vi "ReadButtonUniques.vi"(8 "Error In":errorcluster, 11 "object in":refnum<class "TAFConfiguration.lvclass">) -> (0 "Error Out":errorcluster, 2 "ButtonUniques":T1, 3 "object out":refnum<class "TAFConfiguration.lvclass">)   [LabVIEW 2021, in "TAF Proj Document Type.lvlib" / "TAFConfiguration.lvclass"]
uses:
  <vilib>/Wovalab/AntiDoc/Document Type/Add-ons/LabVIEW TAF Project/TAFConfiguration/TAFConfiguration.lvclass
  <vilib>/Wovalab/AntiDoc/Document Type/Add-ons/LabVIEW TAF Project/TAFConfiguration/TAFConfiguration.lvclass/TAFConfiguration.ctl
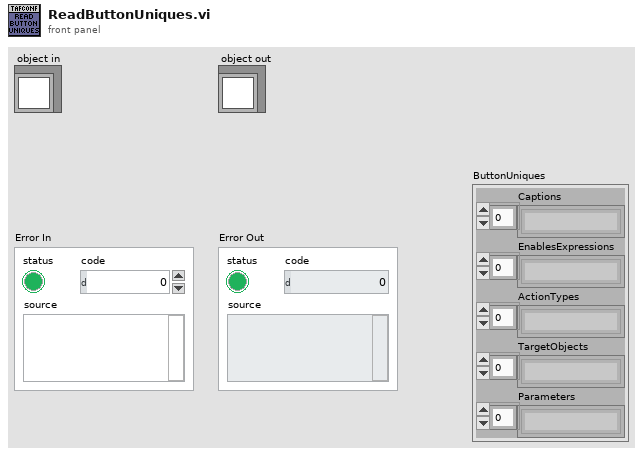
[diagram p1: front panel]
types:
  T1 = cluster{"Captions":string[], "EnablesExpressions":string[], "ActionTypes":string[], "TargetObjects":string[], "Parameters":string[]}
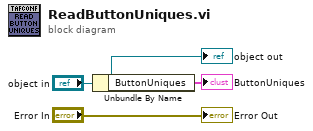
[diagram p0: block diagram]
diagram:
  n1 = Unbundle By Name("object in") -> ("ButtonUniques"=→"ButtonUniques":T1)
  "Error Out" <- "Error In"
  "object out" <- "object in"
